vi "Add More Options.vi"(8 "error in (no error)":errorcluster, 11 "Toolbar Control in":refnum<class "Toolbar Control.lvclass">) -> (0 "error out":errorcluster, 3 "Toolbar Control out":refnum<class "Toolbar Control.lvclass">)   [LabVIEW 2011, in "Toolbar Control.lvclass"]
doc: "This VI will add the More Options button to the toolbar.\n\n-------------\nDeveloped by Brian Hoover (hooovahh)"
uses:
  Toolbar Control.lvclass
  Toolbar Control.lvclass/Toolbar Control.ctl
  Controls/Button State.ctl
  Controls/Icon Type.ctl
  Controls/Icon Data.ctl
  <vilib>/picture/picture.llb/imagedata.ctl
  <vilib>/Utility/miscctls.llb/LVRectTypeDef.ctl
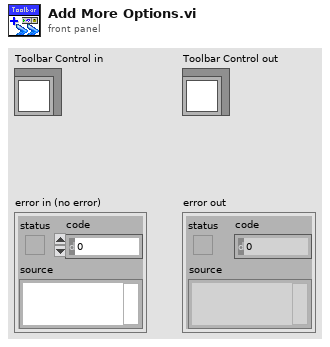
[diagram p1: front panel]
types:
  T1 = typedef "LVRectTypeDef.ctl" = cluster{"Left":i16, "Top":i16, "Right":i16, "Bottom":i16}
  T2 = typedef "Toolbar Control.lvclass/Icon Data.ctl" = cluster{"Original Image Path":path, "Original Image Data":T3, "Scaled Icon":picture, "Button Name":string, "Button State":T4, "Icon Type":T5}
  T3 = typedef "imagedata.ctl" = cluster{"image type":i32, "image depth":i32, "image":u8[], "mask":u8[], "colors":u32[], "Rectangle":cluster{"left":i16, "top":i16, "right":i16, "bottom":i16}}
  T4 = typedef "Toolbar Control.lvclass/Button State.ctl" = enum8{"Enabled", "Disabled", "Disabled and Grayed Out"}
  T5 = typedef "Icon Type.ctl" = enum16{"Normal Icon", "Separator Icon", "More Options"}
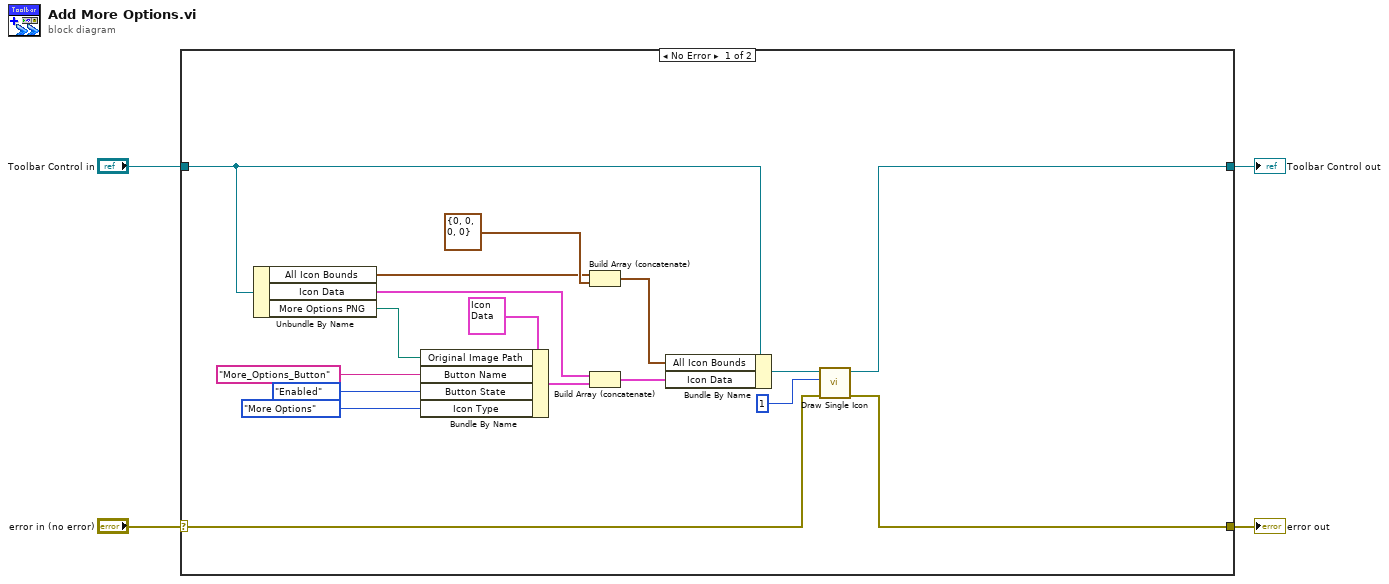
[diagram p0: block diagram]
diagram:
  n1 = case shown="No Error" "error in (no error)" {
    selector: "error in (no error)" -> [w10 w23]
    tunnel: [w9 w23] -> w3
    tunnel: [w8 w22] -> w1
    tunnel: "Toolbar Control in" -> [w15 w22]
    frame No Error {
      n2 = Unbundle By Name(w15) -> ("All Icon Bounds"=w7:T1[], "Icon Data"=w6:T2[], "More Options PNG"=w14:path)
      n3 = Bundle By Name(cluster=T2 {"Original Image Path"=path "", "Original Image Data"={"image type"=0, "image depth"=0, "image"=[], "mask"=[], "colors"=[], "Rectangle"={"left"=0, "top"=0, "right"=0, "bottom"=0}}, "Scaled Icon"=bytes[0], "Button Name"="", "Button State"=enum."Enabled", "Icon Type"=enum."Normal Icon"} ("Cluster"), "Original Image Path"=w14, "Button Name"="More_Options_Button" ("Icon Name"), "Button State"=Button_State."Enabled", "Icon Type"=Icon_Type."More Options") -> (w12:T2)
      n4 = Build Array (concatenate)(w7, T1 {"Left"=0, "Top"=0, "Right"=0, "Bottom"=0} ("Icon Bounds")) -> (w20:T1[])
      n5 = Build Array (concatenate)(w6, w12) -> (w19:T2[])
      n6 = Bundle By Name(cluster=w15, "All Icon Bounds"=w20, "Icon Data"=w19) -> (w21:refnum<class "Toolbar Control.lvclass">)
      n7 = call "Draw Single Icon.vi"("error in (no error)"=w10, "Icon Index"=1, "Toolbar Control in"=w21) -> ("error out"=w9:errorcluster, "Toolbar Control out"=w8:refnum<class "Toolbar Control.lvclass">)  [unwired: 7 in]
    }
    frame Error {
    }
  }
  "error out" <- w3
  "Toolbar Control out" <- w1
